vi "Get Variables.vi"(8 "error in (no error)":errorcluster, 11 "Message Popup in":refnum<class "DMM.lvclass">) -> (0 "error out":errorcluster, 2 "Variables":variant, 3 "Message Popup out":refnum<class "DMM.lvclass">)   [LabVIEW 2019, in "DMM.lvclass"]
uses:
  DMM.lvclass
  DMM.lvclass/DMM.ctl
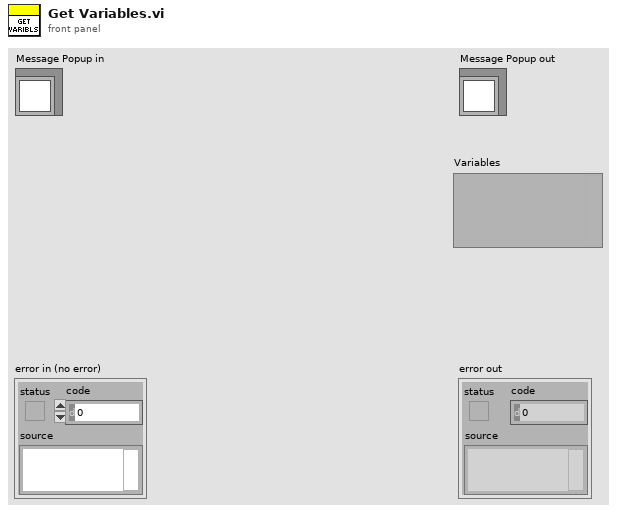
[diagram p1: front panel]
types:
  T1 = typedef "DMM.lvclass/Variables.ctl" = cluster{"instaddress":variant, "instname":string, "channel":string}
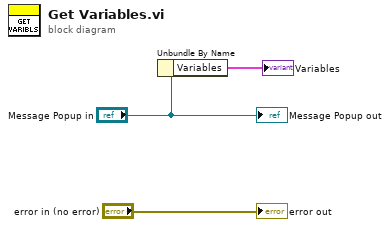
[diagram p0: block diagram]
diagram:
  n1 = Unbundle By Name("Message Popup in") -> ("Variables"=→"Variables":T1)
  "error out" <- "error in (no error)"
  "Message Popup out" <- "Message Popup in"
